vi "remove pre post build from project.vi"(8 "error in (no error)":errorcluster, 11 "Builder in":refnum<class "Builder.lvclass">) -> (0 "error out":errorcluster, 3 "Builder out":refnum<class "Builder.lvclass">)   [LabVIEW 2024, in "Builder.lvclass"]
doc: "If the reference is valid, removes the pre and post build action vis from project"
uses:
  builders/parent/Builder.lvclass
  builders/parent/Builder.lvclass/Builder.ctl
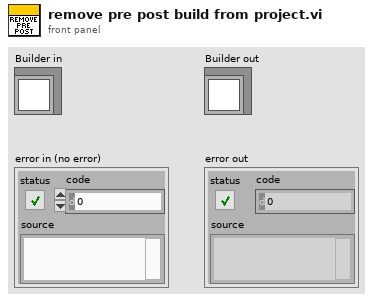
[diagram p1: front panel]
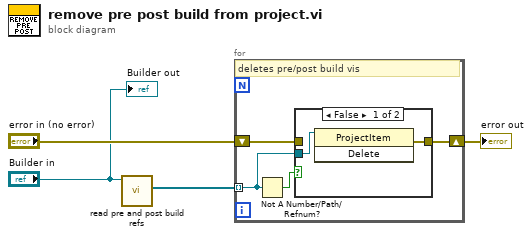
[diagram p0: block diagram]
diagram:
  n1 = call "read pre and post build refs .vi"("Builders in"="Builder in") -> ("pre and post build refs"=w2:refnum<vi>[])  [unwired: 10 in]
  n2 = for {
    tunnel: w2 -> [w6] mode=indexing
    shift-right: [w7] -> w4
    shift-left: "error in (no error)" -> [w8]
    # "deletes pre/post build vis"
    n3 = Not A Number/Path/Refnum?(number/path/refnum=w6) -> (NaN/Path/Refnum?=w5:bool)
    n4 = case shown="False" w5 {
      tunnel: w8 -> [_ w11]
      tunnel: w6 -> [w10 _]
      tunnel: [w9 w11] -> w7
      frame False {
        n5 = invoke class="ProjectItem" method="Delete"(reference=w10) -> (error out=w9:errorcluster)  [unwired: 2 in, 2 out]
      }
      frame True {
      }
    }
  }
  "error out" <- w4
  "Builder out" <- "Builder in"
